vi "min_mark.vi"(9 "element in":T1=255, 10 "square in":i32=5, 11 "pieceOfWorld in in":T2[][](array[typedef])) -> (1 "row 2":i32, 2 "column 2":i32, 3 "Boolean":bool)   [LabVIEW 2015, in "PolyVIEW.lvclass"]
uses:
  PolyVIEW.lvclass
  actors/world/typedefs/worldCell_cluster.ctl
  actors/world/typedefs/markValue_cluster.ctl
  actors/world/typedefs/markValue.ctl
  actors/world/typedefs/markVolume.ctl
  actors/world/typedefs/amountOfFood.ctl
  actors/world/typedefs/anthillType_enum.ctl
  actors/world/world.lvlib
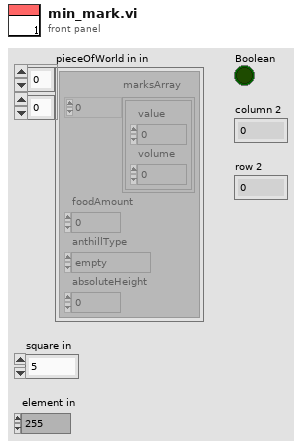
[diagram p1: front panel]
types:
  T1 = typedef "world.lvlib/markValue.ctl" = u8
  T2 = typedef "world.lvlib/worldCell_cluster.ctl" = cluster{"marksArray":T3[], "foodAmount":T5, "anthillType":T6, "absoluteHeight":u8}
  T3 = typedef "world.lvlib/markValue_cluster.ctl" = cluster{"value":T1, "volume":T4}
  T4 = typedef "world.lvlib/markVolume.ctl" = u16
  T5 = typedef "world.lvlib/amountOfFood.ctl" = i32
  T6 = typedef "world.lvlib/anthillType_enum.ctl" = enum16{"empty", "own", "rival"}
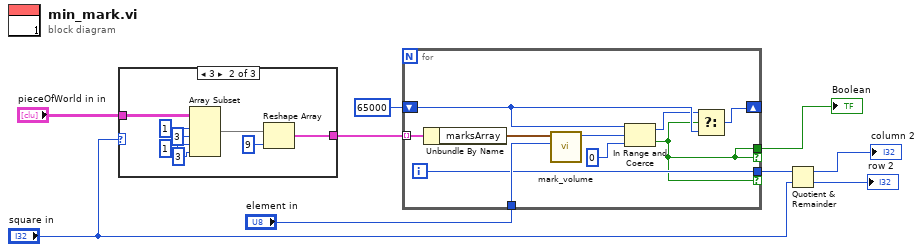
[diagram p0: block diagram]
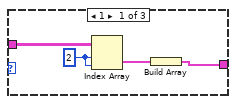
[diagram p2: hidden frame]
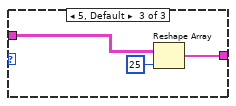
[diagram p3: hidden frame]
diagram:
  n1 = case shown="3" "square in" {
    tunnel: "pieceOfWorld in in" -> [w13 w19 w22]
    tunnel: [w10 w18 w23] -> w7
    frame 1 {
      w12 = 2 ("index (row)")
      n2 = Index Array(array=w13, index (row)=w12, index (col)=w12) -> (element=w11:T2)
      n3 = Build Array(w11) -> (w10:T2[])
    }
    frame 3 {
      n4 = Array Subset(array=w19, index (row)=1 ("index"), length (row)=3 ("length"), index (col)=1 ("index"), length (col)=3 ("length")) -> (w20:T2[][])
      n5 = Reshape Array(w20, 9 ("dimension size")) -> (w18:T2[])
    }
    frame 5, Default {
      n6 = Reshape Array(w22, 25 ("dimension size")) -> (w23:T2[])
    }
  }
  n7 = for {
    tunnel: w7 -> [w34] mode=indexing
    tunnel: "element in" -> [w32]
    shift-right: [w27] -> _
    shift-left: 65000 -> [w28]
    tunnel: [w31] -> w2 if=w25
    tunnel: [w25] -> w9 if=w25
    i -> [w31]
    n8 = Unbundle By Name(w34) -> ("marksArray"=w33:T3[])
    n9 = call "mark_volume.vi"("element"=w32, "marksArray"=w33) -> ("volume"=w30:T4)  [unwired: 9 in]
    n10 = In Range and Coerce(upper limit=w28, x=w30, lower limit=T4 0) -> (coerced(x)=w26:i32, In Range?=w25:bool)
    n11 = Select(t=w26, s=w25, f=w28) -> (s? t:f=w27:i32)
  }
  "Boolean" <- w9
  n12 = Quotient & Remainder(x=w2, y="square in") -> (x-y*floor(x/y)=→"column 2":i32, floor(x/y)=→"row 2":i32)
